vi "BRig_dataExp_I_anySelect.vi"() -> (2 "output_I_anySelect":i32)   [LabVIEW 2014]
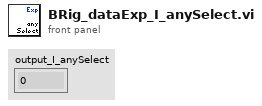
[diagram p1: front panel]
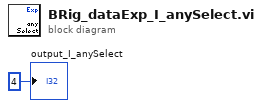
[diagram p0: block diagram]
diagram:
  "output_I_anySelect" <- 4 ("output_iBlock")
